vi "GUID Generator.vi"() -> (3 "GUID":string)   [LabVIEW 2020, in "Custom Device Template Tool.lvlib"]
uses:
  <vilib>/NI VeriStand/Custom Device Tools/Custom Device Template Tool/Custom Device Template Tool.lvlib
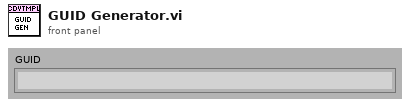
[diagram p1: front panel]
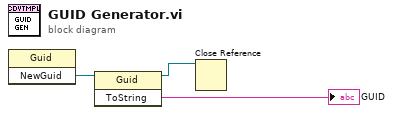
[diagram p0: block diagram]
diagram:
  n1 = invoke class="Guid" method="NewGuid"() -> ("NewGuid"=w3:refnum<k24>)  [unwired: 3 in, 2 out]
  n2 = invoke class="Guid" method="ToString"(reference=w3) -> (reference out=w1:refnum<k24>, "ToString"=→"GUID":string)  [unwired: 2 in, 1 out]
  n3 = Close Reference(reference=w1) -> ()  [unwired: 1 in, 1 out]
